vi "Navigation_Main_r2.2.vi"() -> ()   [LabVIEW 2015]
uses:
  <vilib>/myRIO/Instrument Drivers/Onboard IO/PWM/typedefs/PWM Reference.ctl
  <vilib>/myRIO/Common/Instrument Driver Framework/Utilities/typedefs/myRIO Generic Hardware Reference.ctl
  <vilib>/myRIO/Common/Instrument Driver Framework/Utilities/typedefs/Hardware Version Enum.ctl
  <vilib>/myRIO/Common/Instrument Driver Framework/Utilities/typedefs/myRIO v1.0 Reference.ctl
  <vilib>/myRIO/Common/Instrument Driver Framework/Utilities/typedefs/Generic FPGA Reference.ctl
  <vilib>/myRIO/Common/Instrument Driver Framework/myRIO v1.0/PWM/typedefs/PWM Channels Enum.ctl
  <vilib>/myRIO/Instrument Drivers/Onboard IO/PWM/typedefs/PWM Configuration.ctl
  <vilib>/userdefined/High Color/nirio_resource_hc.ctl
  <vilib>/myRIO/Common/Instrument Driver Framework/myRIO v1.0/PWM/vis/myRIO v1.1 Open PWM.vi
  <vilib>/myRIO/Common/Instrument Driver Framework/Utilities/vis/Validate Channels.vi
  <vilib>/myRIO/Common/Instrument Driver Framework/myRIO v1.0/PWM/vis/myRIO v1.0 Reserve PWM.vi
  <vilib>/myRIO/Common/Instrument Driver Framework/myRIO v1.0/PWM/vis/myRIO v1.0 Build MUX Configuration PWM.vi
  <vilib>/myRIO/Common/Instrument Driver Framework/myRIO v1.0/Resource Manager/vis/myRIO v1.0 Reserve Channel List.vi
  <vilib>/myRIO/Common/Instrument Driver Framework/myRIO v1.0/Resource Manager/vis/myRIO v1.0 Create Configuration List.vi
  <vilib>/myRIO/Common/Instrument Driver Framework/myRIO v1.0/Resource Manager/vis/myRIO v1.0 Reserve Channel.vi
  <vilib>/myRIO/Common/Instrument Driver Framework/myRIO v1.0/Resource Manager/vis/myRIO v1.0 Unreserve Channel.vi
  <vilib>/myRIO/Common/Instrument Driver Framework/myRIO v1.0/Resource Manager/vis/myRIO v1.0 Build Mutex Name.vi
  <vilib>/FPGAPlugInAG/myRIO-1900/niLvFpga_Open_myRIO-1900.vi
  <vilib>/rvi/interface/common/dynamic/niFpgaDynamicAddResources.vi
  <vilib>/myRIO/Common/Instrument Driver Framework/Utilities/vis/FPGA Ref Manager.vi
  <vilib>/Utility/error.llb/Error Cluster From Error Code.vi
  <vilib>/myRIO/Common/Instrument Driver Framework/Utilities/vis/Ref Counter.vi
  <vilib>/rvi/errors/niLvFpgaAdjustHostInterfaceError.vi
  <vilib>/Utility/VariantDataType/GetNumericInfo.vi
  <vilib>/myRIO/Common/Instrument Driver Framework/myRIO v1.0/myRIO v1.1 Open.vi
  <vilib>/myRIO/Common/Instrument Driver Framework/Utilities/vis/IO Manager.vi
  <vilib>/myRIO/Common/Instrument Driver Framework/Utilities/vis/Configuration Manager.vi
  <vilib>/myRIO/Common/Instrument Driver Framework/myRIO v1.0/Resource Manager/vis/myRIO v1.0 Configure IO.vi
  <vilib>/myRIO/Common/Instrument Driver Framework/myRIO v1.0/myRIO v1.0 Close.vi
  <vilib>/myRIO/Common/Instrument Driver Framework/myRIO v1.0/PWM/vis/myRIO v1.0 Write PWM.vi
  <vilib>/addons/control/pid/pid.llb/PID (DBL).vi
  <vilib>/rvi/interface/nirviOpenFPGA/nirviOpenFPGA.xnode
  Navi/E/FPGA Bitfiles/NavigationProjec_FPGATarget2_FPGAMainNavigati_PWPHW8gwDxI.lvbitx
  <vilib>/rvi/interface/nirviReadWriteControl/nirviReadWriteControl.xnode
  <vilib>/myRIO/Instrument Drivers/Onboard IO/PWM/vis/myRIO PWM Open.xnode
  <vilib>/myRIO/Instrument Drivers/Onboard IO/PWM/PWM.lvlib
  <vilib>/myRIO/Instrument Drivers/Utilities/Utilities.lvlib
  NiFpgaLv.dll
  <vilib>/rvi/interface/Simulation/niFpgaSimulationCallBeginRW.vi
  <vilib>/addons/control/pid/NI_PID_pid.lvlib
panel:
  out "Navigation\nCurrent \nAngle":dbl
  out "Navigation\nCurrent y\nPosition":dbl
  out "Navigation\nCurrent X\nPosition":dbl
  out "x+y":dbl
  out "angle command":dbl
  in  "y goal":dbl format="%#_13g"
  out "current angle":dbl
  in  "initial angle":dbl format="%#_13g"
  out "cout per foot":dbl
  out "x/y":dbl
  out "scale":dbl=1.0
  in  "x goal":dbl=10.0
  in  "L Desired Input Velocity (ft/s) 4":dbl(knob) scale=-4.0..4.0
  out "x position 5":dbl
  in  "R Desired Input Velocity (ft/s) 5":dbl(knob) scale=-4.0..4.0
  in  "R Desired Input Velocity (ft/s) 4":dbl(knob) scale=-4.0..4.0
  in  "L Desired Input Velocity (ft/s) 3":dbl(knob) scale=-4.0..4.0
  in  "R Desired Input Velocity (ft/s) 3":dbl(knob) scale=-4.0..4.0
  in  "L Desired Input Velocity (ft/s) 2":dbl(knob) scale=-4.0..4.0
  in  "R Desired Input Velocity (ft/s) 2":dbl(knob) scale=-4.0..4.0
  in  "L Desired Input Velocity (ft/s)":dbl(knob) scale=-4.0..4.0
  out "left":dbl
  out "right":dbl
  out "actual pwm 2":dbl
  in  "stop 3":bool
  out "left pwm":dbl(graph)
  out "dt out (s) 3":dbl format="%.3f"
  in  "output range 3":cluster{"output high":dbl, "output low":dbl}={"output high"=0.13333, "output low"=-0.13333} {"output low" format="%.6f"; "output high" format="%.5f"}
  in  "PID gains 3":T1={"proportional gain (Kc)"=0.002, "integral time (Ti, min)"=7e-07, "derivative time (Td, min)"=0.0} {"derivative time (Td, min)" format="%.8f"; "integral time (Ti, min)" format="%.8f"; "proportional gain (Kc)" format="%.8f"}
  out "desired pwm 2":dbl
  out "feedback 2":dbl
  out ".not. x? 3":bool
  out "Elapsed Time (s) 2":dbl caption="Elapsed Time (s)"
  out "x traveled 2":dbl
  out "y traveled 2":dbl
  out "avg right":dbl
  out "avg left":dbl
  out "psi dot":dbl
  out "distance traveled 2":dbl
  out "y dot 2":dbl
  out "x dot 2":dbl
  out "x position":dbl
  out "y position":dbl
  out "reset x y 2":dbl
  out "Tick Count(mSec) 2":u32 caption="Tick Count(mSec)"
  in  "start y 2":dbl=3.0
  in  "start x 2":dbl=1.0
  in  "start y":dbl=3.0
  in  "start x":dbl=1.0
  in  "Encoder Reset 2":bool
  out "actual pwm":dbl
  in  "stop 2":bool
  out "right pwm":dbl(graph)
  out "dt out (s) 2":dbl format="%.3f"
  in  "output range 2":cluster{"output high":dbl, "output low":dbl}={"output high"=0.13333, "output low"=-0.13333} {"output low" format="%.6f"; "output high" format="%.5f"}
  in  "PID gains 2":T1={"proportional gain (Kc)"=0.002, "integral time (Ti, min)"=7e-07, "derivative time (Td, min)"=0.0} {"derivative time (Td, min)" format="%.8f"; "integral time (Ti, min)" format="%.8f"; "proportional gain (Kc)" format="%.8f"}
  out "desired pwm":dbl
  out "feedback":dbl
  out ".not. x? 2":bool
  out "Elapsed Time (s)":dbl
  out "LF Rot Velocity (rot/s)":dbl
  out "LM Rot Velocity (rot/s)":dbl
  out "LR Rot Velocity (rot/s)":dbl
  out "RR Rot Velocity (rot/s)":dbl
  out "RM Linear Velocity (rot/s)":dbl
  out "RF Linear Velocity (rot/s)":dbl
  in  "Encoder Reset":bool
  out "SYS.SELECTA":u8 format="%08b"
  out "ENC.B_c.CNTR":i32
  out "ENC.B_b.CNTR":i32
  out "ENC.B_a.CNTR":i32
  out "ENC.A_c.CNTR":i32
  out "ENC.A_b.CNTR":i32
  out "ENC.A_a.CNTR":i32
  in  "R Min Linear Velocity (ft/s)":dbl=-2.0 format="%#_13g"
  in  "R Max Linear Velocity (ft/s)":dbl=2.0 format="%#_13g"
  in  "L Min Linear Velocity (ft/s)":dbl=-2.0 format="%#_13g"
  in  "L Max Linear Velocity (ft/s)":dbl=2.0 format="%#_13g"
  out "Current Rot Velocity (rot/s)":T2(graph)
  # "Motor Control Parameters"
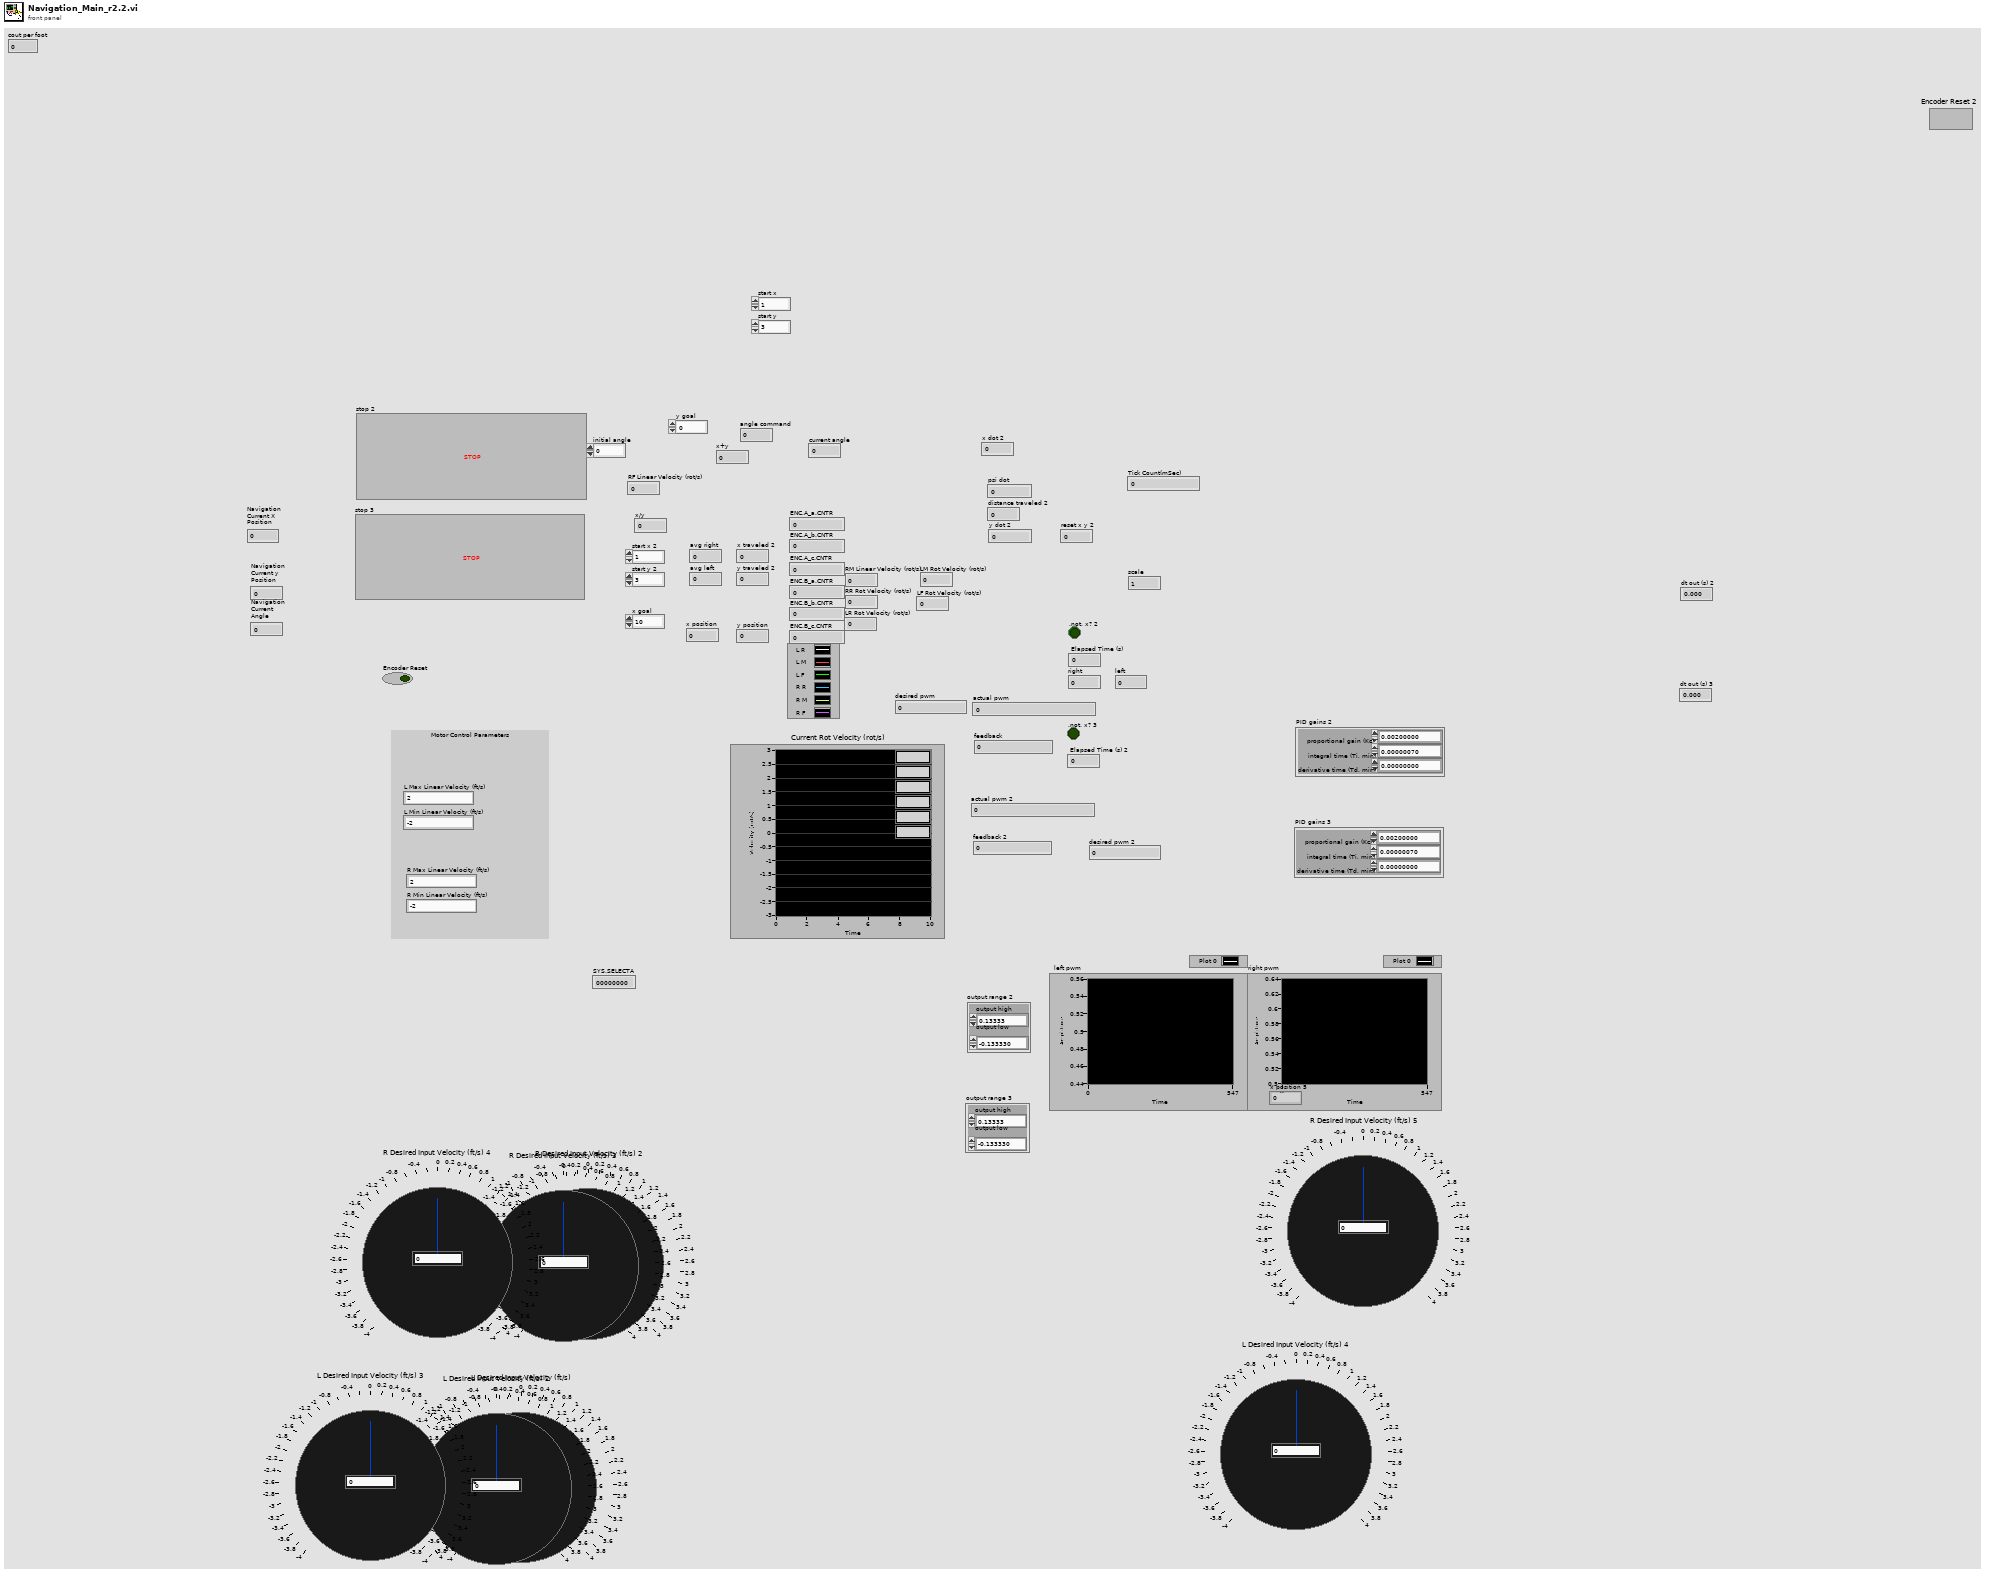
[diagram p1: front panel]
types:
  T1 = cluster{"proportional gain (Kc)":dbl, "integral time (Ti, min)":dbl, "derivative time (Td, min)":dbl}
  T2 = cluster{"Rotational Velocity (RPS)":dbl, "Rotational Velocity (RPS)":dbl, "Rotational Velocity (RPS)":dbl, "Rotational Velocity (RPS)":dbl, "Rotational Velocity (RPS)":dbl, "Rotational Velocity (RPS)":dbl}
  T3 = typedef "nirio_resource_hc.ctl" = tag
  T4 = typedef "Hardware Version Enum.ctl" = enum16{"Unknown", "myRIO-1900", "myRIO-1950", "roboRIO"}
  T5 = typedef "PWM.lvlib/PWM Reference.ctl" = cluster{"myRIO Reference":T6, "PWM Channels Enum":T9, "PWM Configuration":T10}
  T6 = typedef "myRIO Generic Hardware Reference.ctl" = cluster{"myRIO Model":T4, "myRIO Hardware Reference":T7}
  T7 = typedef "myRIO v1.0 Reference.ctl" = cluster{"Generic FPGA Reference":T8, "Allow multiple opens":bool}
  T8 = typedef "Generic FPGA Reference.ctl" = refnum<k20>
  T9 = typedef "PWM Channels Enum.ctl" = enum16{"Not Connected", "C/PWM0", "C/PWM1", "A/PWM0", "A/PWM1", "A/PWM2", "B/PWM0", "B/PWM1", "B/PWM2", "PWM/PWM0", "PWM/PWM1", "PWM/PWM2", "PWM/PWM3", "PWM/PWM4", "PWM/PWM5", "PWM/PWM6", "PWM/PWM7", "PWM/PWM8", "PWM/PWM9"}
  T10 = typedef "PWM.lvlib/PWM Configuration.ctl" = cluster{"Frequency":dbl, "Duty Cycle":dbl}
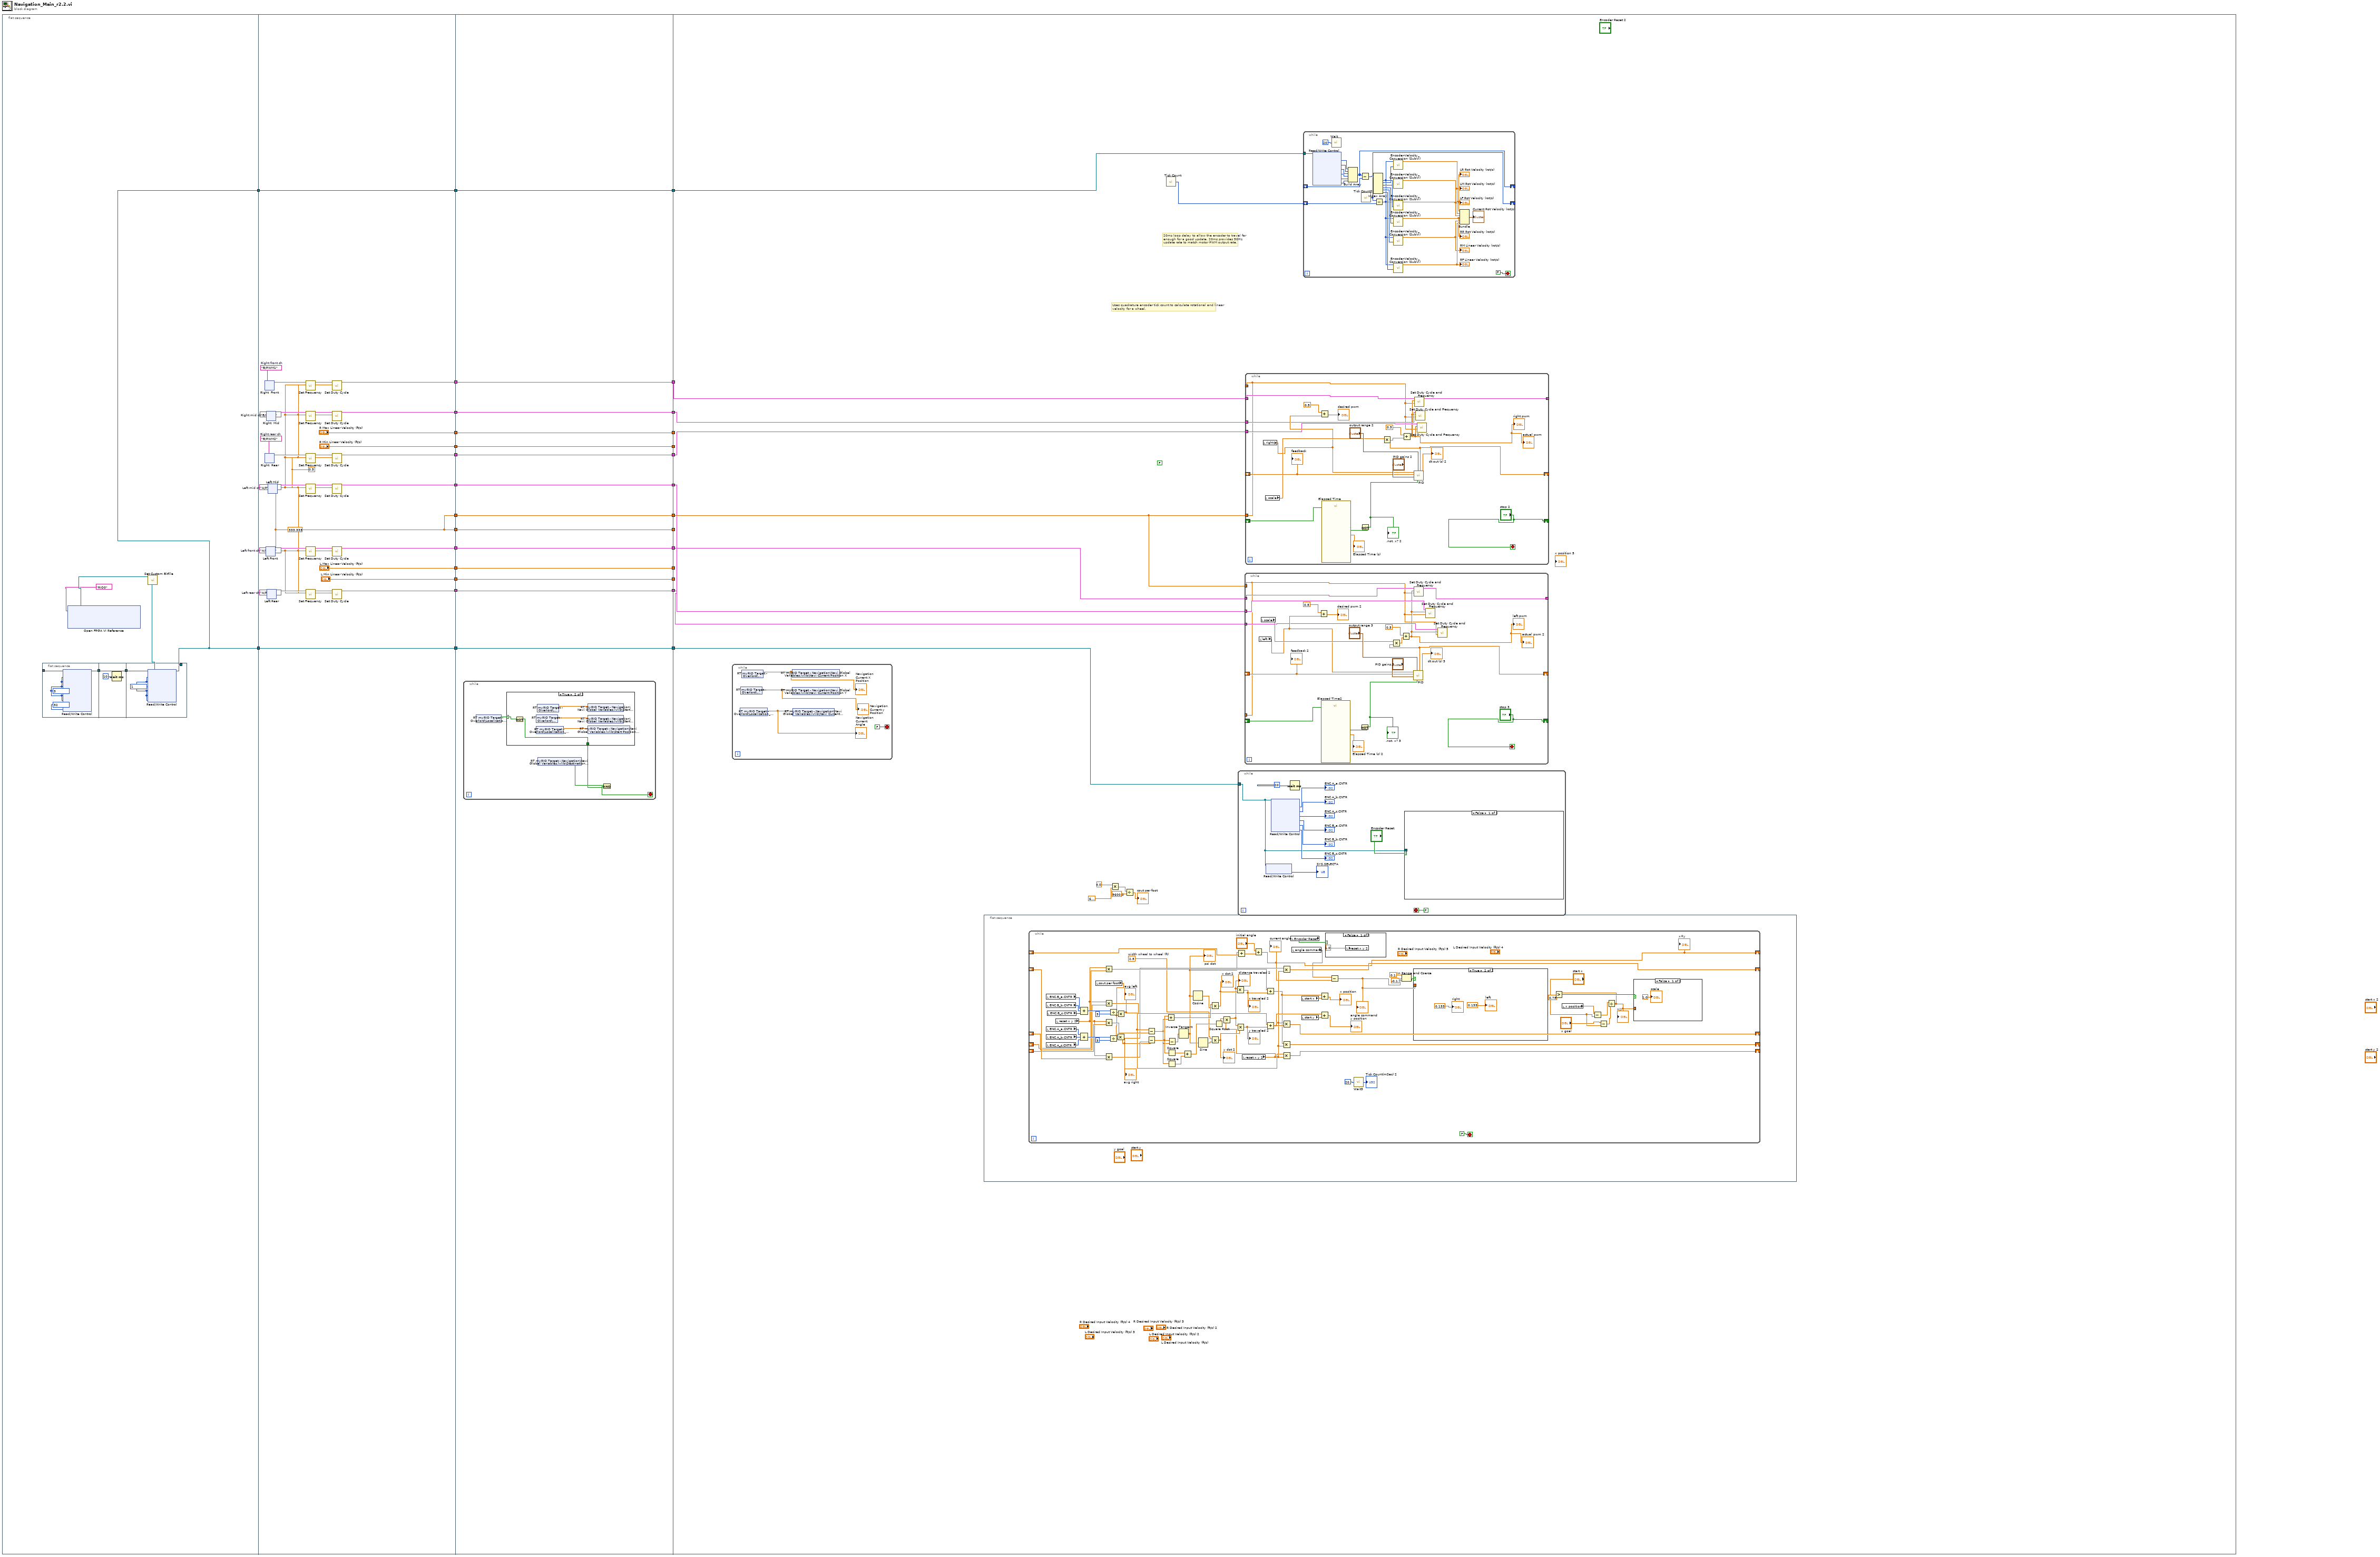
[diagram p0: block diagram]
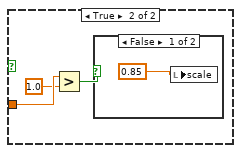
[diagram p3: hidden frame]
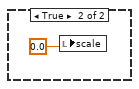
[diagram p4: hidden frame]
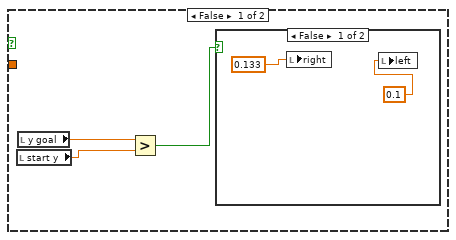
[diagram p5: hidden frame]
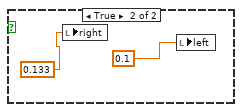
[diagram p6: hidden frame]
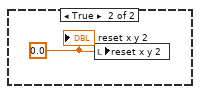
[diagram p7: hidden frame]
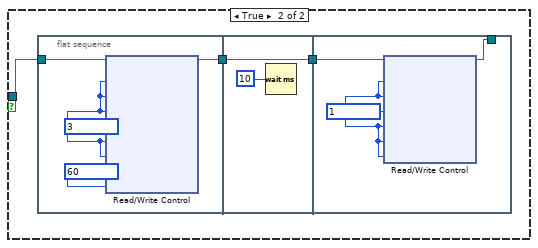
[diagram p8: hidden frame]
diagram:
  n1 = flat-sequence {
    tunnel: [w33] -> w30
    tunnel: [w33] -> w29
    tunnel: [w46] -> w28
    tunnel: [w61] -> w26
    tunnel: [w57] -> w24
    tunnel: [w56] -> w22
    tunnel: [w55] -> w20
    tunnel: [w54] -> w18
    tunnel: [w53] -> w16
    tunnel: ["L Max Linear Velocity (ft/s)"] -> w14
    tunnel: ["L Min Linear Velocity (ft/s)"] -> w12
    tunnel: ["R Max Linear Velocity (ft/s)"] -> w10
    tunnel: ["R Min Linear Velocity (ft/s)"] -> w8
    tunnel: [w48] -> w6
    tunnel: w30 -> [w47]
    tunnel: [w47] -> w4
    tunnel: w29 -> [w48]
    tunnel: [w46] -> w2
    tunnel: w28 -> [w187]
    tunnel: [w187] -> w27
    tunnel: w26 -> [w186]
    tunnel: [w186] -> w25
    tunnel: w24 -> [w185]
    tunnel: [w185] -> w23
    tunnel: w22 -> [w184]
    tunnel: [w184] -> w21
    tunnel: w20 -> [w183]
    tunnel: [w183] -> w19
    tunnel: w18 -> [w182]
    tunnel: [w182] -> w17
    tunnel: w16 -> [w181]
    tunnel: [w181] -> w15
    tunnel: w14 -> [w180]
    tunnel: [w180] -> w13
    tunnel: w12 -> [w179]
    tunnel: [w179] -> w11
    tunnel: w10 -> [w178]
    tunnel: [w178] -> w9
    tunnel: w8 -> [w177]
    tunnel: [w177] -> w7
    tunnel: w6 -> [w176]
    tunnel: [w176] -> w5
    tunnel: w4 -> [w175]
    tunnel: [w175] -> w3
    tunnel: w2 -> [w174]
    tunnel: [w174] -> w1
    tunnel: w27 -> [_]
    tunnel: w25 -> [w202]
    tunnel: w23 -> [w208]
    tunnel: w21 -> [w205]
    tunnel: w19 -> [w204]
    tunnel: w17 -> [w203]
    tunnel: w15 -> [w207]
    tunnel: w13 -> [_]
    tunnel: w11 -> [_]
    tunnel: w9 -> [_]
    tunnel: w7 -> [_]
    tunnel: w5 -> [w210]
    tunnel: w3 -> [w209]
    tunnel: w1 -> [w206]
    frame #0 {
      n2 = flat-sequence {
        tunnel: w34 -> [w39]
        tunnel: [w37] -> w36
        tunnel: w36 -> [w41]
        tunnel: [w41] -> w35
        tunnel: w35 -> [w44]
        tunnel: [w43] -> w33
        frame #0 {
          w38 = u8 32 ("SYS.SELECTA")
          w40 = u8 3 ("ENC.B_c.CNFG")
          n3 = xnode "Read/Write Control"("FPGA VI Reference In"=w39, "ENC.A_a.CNFG"=w40, "ENC.A_b.CNFG"=w40, "ENC.A_c.CNFG"=w40, "ENC.B_a.CNFG"=w40, "ENC.B_b.CNFG"=w40, "ENC.B_c.CNFG"=w40, "SYS.SELECTA"=w38, "SYS.SELECTB"=w38) -> ("FPGA VI Reference Out"=w37:refnum<k20>)  [unwired: 1 in, 1 out]
        }
        frame #1 {
          n4 = Wait (ms)(milliseconds to wait=u32 10) -> ()  [unwired: 1 out]
        }
        frame #2 {
          w45 = u8 1 ("ENC.B_c.CNFG")
          n5 = xnode "Read/Write Control"("FPGA VI Reference In"=w44, "ENC.A_a.CNFG"=w45, "ENC.A_b.CNFG"=w45, "ENC.A_c.CNFG"=w45, "ENC.B_a.CNFG"=w45, "ENC.B_b.CNFG"=w45, "ENC.B_c.CNFG"=w45) -> ("FPGA VI Reference Out"=w43:refnum<k20>)  [unwired: 1 in, 1 out]
        }
      }
      n6 = xnode "Open FPGA VI Reference"("resource name"=tag "RIO0") -> ("FPGA VI Reference Out"=w32:refnum<k20>)  [unwired: 1 in, 1 out]
      n7 = call <vilib>:"Set Custom Bitfile.vi"("Custom FPGA Reference In"=w32) -> ("Custom FPGA Reference Out"=w34:refnum<k20>)  [unwired: 9 in, 1 out]
    }
    frame #1 {
      w58 = 0.5 ("Duty Cycle")
      w46 = 333.333 ("Frequency [Hz]")
      w72 = tag "B/PWM2"  # Right rear ch
      w73 = tag "B/PWM0"  # Right mid ch
      w74 = tag "B/PWM1"  # Right front ch
      w75 = tag "A/PWM2"  # Left rear ch
      w76 = tag "A/PWM1"  # Left mid ch
      w77 = tag "A/PWM0"  # Left front ch
      n8 = xnode "Right  Front"("Channel Name"=w74) -> ("PWM Ref Out"=w68:T5)  [unwired: 2 in, 1 out]
      n9 = xnode "Right  Rear"("Channel Name"=w72) -> ("PWM Ref Out"=w66:T5)  [unwired: 2 in, 1 out]
      n10 = xnode "Left Front"("Channel Name"=w77) -> ("PWM Ref Out"=w71:T5)  [unwired: 2 in, 1 out]
      n11 = xnode "Right  Mid"("Channel Name"=w73) -> ("PWM Ref Out"=w67:T5)  [unwired: 2 in, 1 out]
      n12 = xnode "Left Rear"("Channel Name"=w75) -> ("PWM Ref Out"=w69:T5)  [unwired: 2 in, 1 out]
      n13 = xnode "Left Mid"("Channel Name"=w76) -> ("PWM Ref Out"=w70:T5)  [unwired: 2 in, 1 out]
      n14 = call <vilib>:"Set Frequency.vi"("Frequency [Hz]"=w46, "PWM Ref In"=w68) -> ("PWM Ref Out"=w62:T5)  [unwired: 7 in, 1 out]
      n15 = call <vilib>:"Set Frequency.vi"("Frequency [Hz]"=w46, "PWM Ref In"=w67) -> ("PWM Ref Out"=w63:T5)  [unwired: 7 in, 1 out]
      n16 = call <vilib>:"Set Frequency.vi"("Frequency [Hz]"=w46, "PWM Ref In"=w66) -> ("PWM Ref Out"=w64:T5)  [unwired: 7 in, 1 out]
      n17 = call <vilib>:"Set Frequency.vi"("Frequency [Hz]"=w46, "PWM Ref In"=w70) -> ("PWM Ref Out"=w59:T5)  [unwired: 7 in, 1 out]
      n18 = call <vilib>:"Set Frequency.vi"("Frequency [Hz]"=w46, "PWM Ref In"=w71) -> ("PWM Ref Out"=w65:T5)  [unwired: 7 in, 1 out]
      n19 = call <vilib>:"Set Frequency.vi"("Frequency [Hz]"=w46, "PWM Ref In"=w69) -> ("PWM Ref Out"=w60:T5)  [unwired: 7 in, 1 out]
      n20 = call <vilib>:"Set Duty Cycle.vi"("Duty Cycle"=w58, "PWM Ref In"=w62) -> ("PWM Ref Out"=w57:T5)  [unwired: 7 in, 1 out]
      n21 = call <vilib>:"Set Duty Cycle.vi"("Duty Cycle"=w58, "PWM Ref In"=w63) -> ("PWM Ref Out"=w56:T5)  [unwired: 7 in, 1 out]
      n22 = call <vilib>:"Set Duty Cycle.vi"("Duty Cycle"=w58, "PWM Ref In"=w64) -> ("PWM Ref Out"=w55:T5)  [unwired: 7 in, 1 out]
      n23 = call <vilib>:"Set Duty Cycle.vi"("Duty Cycle"=w58, "PWM Ref In"=w59) -> ("PWM Ref Out"=w54:T5)  [unwired: 7 in, 1 out]
      n24 = call <vilib>:"Set Duty Cycle.vi"("Duty Cycle"=w58, "PWM Ref In"=w65) -> ("PWM Ref Out"=w53:T5)  [unwired: 7 in, 1 out]
      n25 = call <vilib>:"Set Duty Cycle.vi"("Duty Cycle"=w58, "PWM Ref In"=w60) -> ("PWM Ref Out"=w61:T5)  [unwired: 7 in, 1 out]
    }
    frame #2 {
      n26 = while {
        stop <- w190 stop-if-true
        n27 = shared-variable "RT myRIO Target - Overlord\\Localization_Variables_r0.lvlib\\loc_flag"() -> (w189:bool)  [unwired: 1 in, 1 out]
        n28 = case shown="True" w189 {
          selector: w189 -> [_ w194]
          tunnel: [_ w193] -> w188
          frame False {
          }
          frame True {
            n29 = Not(x=w194) -> (.not. x?=w193:bool)
            n30 = shared-variable "RT myRIO Target - Overlord\\Localization_Variables_r0.lvlib\\loc_theta"() -> (w192:dbl)  [unwired: 1 in, 1 out]
            n31 = shared-variable "RT myRIO Target - Overlord\\Localization_Variables_r0.lvlib\\loc_y"() -> (w195:dbl)  [unwired: 1 in, 1 out]
            n32 = shared-variable "RT myRIO Target - Overlord\\Localization_Variables_r0.lvlib\\loc_x"() -> (w196:dbl)  [unwired: 1 in, 1 out]
            n33 = shared-variable "RT myRIO Target - Navigation\\Navi Global Variables.lvlib\\Start Position X"(w196) -> ()  [unwired: 1 in, 1 out]
            n34 = shared-variable "RT myRIO Target - Navigation\\Navi Global Variables.lvlib\\Start Position Y"(w195) -> ()  [unwired: 1 in, 1 out]
            n35 = shared-variable "RT myRIO Target - Navigation\\Navi Global Variables.lvlib\\Start Position Angle"(w192) -> ()  [unwired: 1 in, 1 out]
          }
        }
        n36 = shared-variable "RT myRIO Target - Navigation\\Navi Global Variables.lvlib\\Destination Reached"() -> (w191:bool)  [unwired: 1 in, 1 out]
        n37 = And(x=w191, y=w188) -> (x .and. y?=w190:bool)
      }
    }
    frame #3 {
      (unwired) FALSE
      # "Uses quadrature encoder tick count to calculate rotational and linear velocity for a wheel."
      # "20ms loop delay to allow the encoder to travel far enough for a good update. 20ms provides 50Hz update rate to match motor PWM output rate."
      n38 = while {
        stop <- FALSE stop-if-true
        n39 = shared-variable "RT myRIO Target - Overlord\\Localization_Variables_r0.lvlib\\loc_theta"() -> (w212:dbl)  [unwired: 1 in, 1 out]
        "Navigation\nCurrent \nAngle" <- w212
        n40 = shared-variable "RT myRIO Target - Overlord\\Localization_Variables_r0.lvlib\\loc_y"() -> (w213:dbl)  [unwired: 1 in, 1 out]
        "Navigation\nCurrent y\nPosition" <- w213
        n41 = shared-variable "RT myRIO Target - Overlord\\Localization_Variables_r0.lvlib\\loc_x"() -> (w214:dbl)  [unwired: 1 in, 1 out]
        "Navigation\nCurrent X\nPosition" <- w214
        n42 = shared-variable "RT myRIO Target - Navigation\\Navi Global Variables.lvlib\\Navi Current Position X"(w214) -> ()  [unwired: 1 in, 1 out]
        n43 = shared-variable "RT myRIO Target - Navigation\\Navi Global Variables.lvlib\\Navi Current Position Y"(w213) -> ()  [unwired: 1 in, 1 out]
        n44 = shared-variable "RT myRIO Target - Navigation\\Navi Global Variables.lvlib\\Navi Current Angle"(w212) -> ()  [unwired: 1 in, 1 out]
      }
      n45 = flat-sequence {
        frame #0 {
          n46 = while {
            shift-right: [w250] -> _
            shift-left: _ -> [w275]
            shift-right: [w247] -> _
            shift-left: _ -> [w274]
            shift-right: [w249] -> _
            shift-left: _ -> [w259]
            shift-right: [w248] -> _
            shift-left: _ -> [w258]
            shift-right: [w224] -> _
            shift-left: _ -> [w228]
            stop <- FALSE stop-if-true
            w221 = 2.5  # width wheel to wheel (ft)
            n47 = local read "ENC.B_a.CNTR"() -> (w280:i32)
            n48 = local read "ENC.B_b.CNTR"() -> (w279:i32)
            n49 = local read "ENC.A_a.CNTR"() -> (w283:i32)
            n50 = local read "ENC.A_b.CNTR"() -> (w282:i32)
            n51 = local read "ENC.A_c.CNTR"() -> (w281:i32)
            n52 = local read "ENC.B_c.CNTR"() -> (w278:i32)
            n53 = local read "reset x y 2"() -> (w246:dbl)
            n54 = Compound Arithmetic op=ADD(w280, w279, w278) -> (w286:i32)
            n55 = Compound Arithmetic op=ADD(w283, w282, w281) -> (w287:i32)
            n56 = local read "cout per foot"() -> (w229:dbl)
            n57 = Multiply(x=w246, y=w258) -> (x*y=w252:dbl)
            n58 = Multiply(x=w246, y=w259) -> (x*y=w253:dbl)
            n59 = Multiply(x=w246, y=w274) -> (x*y=w251:dbl)
            n60 = Multiply(x=w246, y=w275) -> (x*y=w254:dbl)
            n61 = Divide(x=w286, y=3) -> (x/y=w273:dbl)
            n62 = Divide(x=w287, y=3) -> (x/y=w276:dbl)
            n63 = Multiply(x=w229, y=w276) -> (x*y=w230:dbl)
            "avg right" <- w230
            n64 = Multiply(x=w273, y=w229) -> (x*y=w231:dbl)
            "avg left" <- w231
            n65 = Subtract(x=w231, y=w251) -> (x-y=w270:dbl)
            n66 = Subtract(x=w230, y=w254) -> (x-y=w271:dbl)
            n67 = Add(x=w271, y=w270) -> (x+y=w272:dbl)
            n68 = Square(x=w271) -> (x^2=w268:dbl)
            n69 = Square(x=w270) -> (x^2=w269:dbl)
            n70 = Subtract(x=w271, y=w270) -> (x-y=w220:dbl)
            n71 = Inverse Tangent(1:w220) -> (0:w225:dbl)
            "psi dot" <- w225
            n72 = Add(x=w268, y=w269) -> (x+y=w267:dbl)
            n73 = Cosine(x=w225) -> (cos(x)=w265:dbl)
            n74 = Sine(x=w225) -> (sin(x)=w266:dbl)
            n75 = Multiply(x=w272, y=w265) -> (x*y=w263:dbl)
            "x dot 2" <- w263
            n76 = Multiply(x=w221, y=w266) -> (x*y=w264:dbl)
            "y dot 2" <- w264
            n77 = Square Root(x=w267) -> (sqrt(x)=w262:dbl)
            n78 = Add(x=w225, y=w228) -> (x+y=w227:dbl)
            n79 = local read "reset x y 2"() -> (w244:dbl)
            n80 = Multiply(x=w262, y=w244) -> (x*y=w245:dbl)
            "distance traveled 2" <- w245
            n81 = Multiply(x=w245, y=w263) -> (x*y=w261:dbl)
            "x traveled 2" <- w261
            n82 = Multiply(x=w245, y=w264) -> (x*y=w260:dbl)
            "y traveled 2" <- w260
            n83 = Add(x="initial angle", y=w227) -> (x+y=w224:dbl)
            "current angle" <- w224
            "x+y" <- w224
            n84 = Add(x=w252, y=w261) -> (x+y=w223:dbl)
            n85 = Add(x=w253, y=w260) -> (x+y=w255:dbl)
            n86 = Multiply(x=w230, y=w244) -> (x*y=w250:dbl)
            n87 = Multiply(x=w244, y=w255) -> (x*y=w249:dbl)
            n88 = Multiply(x=w223, y=w244) -> (x*y=w248:dbl)
            n89 = Multiply(x=w231, y=w244) -> (x*y=w247:dbl)
            n90 = local read "Encoder Reset"() -> (w243:bool)
            n91 = local read "angle command"() -> (w222:dbl)
            n92 = local read "start x"() -> (w256:dbl)
            n93 = local read "start y"() -> (w257:dbl)
            n94 = Add(x=w223, y=w256) -> (x+y=→"x position":dbl)
            n95 = Add(x=w255, y=w257) -> (x+y=→"y position":dbl)
            n96 = case shown="False" w243 {
              frame False {
                n97 = local write "reset x y 2"(1.0) -> ()
              }
              frame True {
                w305 = 0.0
                n98 = local write "reset x y 2"(w305) -> ()
                "reset x y 2" <- w305
              }
            }
            n99 = Subtract(x=w222, y=w224) -> (x-y=w216:dbl)
            "angle command" <- w216
            n100 = call "Wait3"("Count(mSec)"=u32 20) -> ("Tick Count(mSec)"=→"Tick Count(mSec) 2":u32)
            n101 = In Range and Coerce(upper limit=0.1 ("y"), x=w216, lower limit=-0.1) -> (In Range?=w219:bool)  [unwired: 1 out]
            n102 = case shown="True" w219 {
              tunnel: w216 -> [_ _]
              frame False {
                n103 = local read "start y"() -> (w296:dbl)
                n104 = local read "y goal"() -> (w297:dbl)
                n105 = Greater?(x=w297, y=w296) -> (0:w295:bool)
                n106 = case shown="False" w295 {
                  frame False {
                    n107 = local write "right"(0.133) -> ()
                    n108 = local write "left"(0.1 ("left")) -> ()
                  }
                  frame True {
                    n109 = local write "right"(0.133) -> ()
                    n110 = local write "left"(0.1) -> ()
                  }
                }
              }
              frame True {
                "right" <- 0.133
                "left" <- 0.133
              }
            }
            n111 = local read "x position"() -> (w239:dbl)
            n112 = Subtract(x=w239, y="start x") -> (x-y=w233:dbl)
            n113 = Subtract(x="x goal", y="start x") -> (x-y=w232:dbl)
            n114 = Divide(x=w233, y=w232) -> (x/y=w236:dbl)
            "x/y" <- w236
            n115 = Greater?(x=w236, y=0.75) -> (0:w237:bool)
            n116 = case shown="False" w237 {
              tunnel: w236 -> [_ w292]
              frame False {
                "scale" <- 1.0
              }
              frame True {
                n117 = Greater?(x=w292, y=1.0) -> (0:w290:bool)
                n118 = case shown="False" w290 {
                  frame False {
                    n119 = local write "scale"(0.85) -> ()
                  }
                  frame True {
                    n120 = local write "scale"(0.0) -> ()
                  }
                }
              }
            }
          }
        }
      }
      n121 = Multiply(x=4.0, y=6.283185307179586) -> (x*y=w197:dbl)
      n122 = Divide(x=w197, y=9600.0) -> (x/y=→"cout per foot":dbl)
      n123 = call "Tick Count"() -> ("Tick Count(uSec)"=w211:u32)
      n124 = while {
        tunnel: w210 -> [w350]
        stop <- FALSE stop-if-true
        n125 = xnode "Read/Write Control"("FPGA VI Reference In"=w350) -> ("SYS.SELECTA"=→"SYS.SELECTA":u8)  [unwired: 1 in, 2 out]
        n126 = xnode "Read/Write Control"("FPGA VI Reference In"=w350) -> ("ENC.A_a.CNTR"=→"ENC.A_a.CNTR":u32, "ENC.A_b.CNTR"=→"ENC.A_b.CNTR":u32, "ENC.A_c.CNTR"=→"ENC.A_c.CNTR":u32, "ENC.B_a.CNTR"=→"ENC.B_a.CNTR":u32, "ENC.B_b.CNTR"=→"ENC.B_b.CNTR":u32, "ENC.B_c.CNTR"=→"ENC.B_c.CNTR":u32)  [unwired: 1 in, 2 out]
        n127 = Wait (ms)(milliseconds to wait=u32 20) -> ()  [unwired: 1 out]
        n128 = case shown="False" "Encoder Reset" {
          tunnel: w350 -> [_ w361]
          frame False {
          }
          frame True {
            n129 = flat-sequence {
              tunnel: w361 -> [w366]
              tunnel: [w364] -> w363
              tunnel: w363 -> [w368]
              tunnel: [w368] -> w362
              tunnel: w362 -> [w371]
              tunnel: [w370] -> _
              frame #0 {
                w365 = u8 60 ("SYS.SELECTA")
                w367 = u8 3 ("ENC.B_c.CNFG")
                n130 = xnode "Read/Write Control"("FPGA VI Reference In"=w366, "ENC.A_a.CNFG"=w367, "ENC.A_b.CNFG"=w367, "ENC.A_c.CNFG"=w367, "ENC.B_a.CNFG"=w367, "ENC.B_b.CNFG"=w367, "ENC.B_c.CNFG"=w367, "SYS.SELECTA"=w365, "SYS.SELECTB"=w365) -> ("FPGA VI Reference Out"=w364:refnum<k20>)  [unwired: 1 in, 1 out]
              }
              frame #1 {
                n131 = Wait (ms)(milliseconds to wait=u32 10) -> ()  [unwired: 1 out]
              }
              frame #2 {
                w372 = u8 1 ("ENC.B_c.CNFG")
                n132 = xnode "Read/Write Control"("FPGA VI Reference In"=w371, "ENC.A_a.CNFG"=w372, "ENC.A_b.CNFG"=w372, "ENC.A_c.CNFG"=w372, "ENC.B_a.CNFG"=w372, "ENC.B_b.CNFG"=w372, "ENC.B_c.CNFG"=w372) -> ("FPGA VI Reference Out"=w370:refnum<k20>)  [unwired: 1 in, 1 out]
              }
            }
          }
        }
      }
      n133 = while {
        tunnel: w207 -> [w326]
        tunnel: [w327] -> _
        tunnel: w206 -> [w306]
        shift-right: [w312] -> _
        shift-left: _ -> [w322]
        shift-right: ["stop 3"] -> _
        shift-left: _ -> [w317]
        tunnel: [w306] -> _
        tunnel: w203 -> [w309]
        tunnel: w202 -> [w308]
        stop <- "stop 3" stop-if-true
        n134 = local read "left"() -> (w310:dbl)
        n135 = local read "scale"() -> (w313:dbl)
        n136 = Add(x=0.5, y=w310) -> (x+y=→"desired pwm 2":dbl)
        n137 = call "Elapsed Time2"("Reset"=w317) -> ("Elapsed Time (s)"=→"Elapsed Time (s) 2":dbl, "Time has Elapsed"=w320:bool)  [unwired: 11 in, 6 out]
        n138 = Not(x=w320) -> (.not. x?=w319:bool)
        ".not. x? 3" <- w319
        n139 = call-poly <vilib>:"PID.vi"("reinitialize? (F)"=w319, "output range"="output range 3", "PID gains"="PID gains 3", "process variable"=w322, "setpoint"=w310) -> ("dt out (s)"=→"dt out (s) 3":dbl, "output"=w312:dbl)  [unwired: 5 in]
        n140 = Multiply(x=w313, y=w312) -> (x*y=w311:dbl)
        n141 = Add(x=0.5, y=w311) -> (x+y=w307:dbl)
        "actual pwm 2" <- w307
        "left pwm" <- w307
        n142 = call <vilib>:"Set Duty Cycle and Frequency.vi"("Frequency [Hz]"=w306, "Duty Cycle"=w307, "PWM Ref In"=w326) -> ("PWM Ref Out"=w327:T5)  [unwired: 6 in, 1 out]
        n143 = call <vilib>:"Set Duty Cycle and Frequency.vi"("Frequency [Hz]"=w306, "Duty Cycle"=w307, "PWM Ref In"=w309) -> ()  [unwired: 6 in, 2 out]
        n144 = call <vilib>:"Set Duty Cycle and Frequency.vi"("Frequency [Hz]"=w306, "Duty Cycle"=w307, "PWM Ref In"=w308) -> ()  [unwired: 6 in, 2 out]
        "feedback 2" <- w322
      }
      n145 = while {
        tunnel: w208 -> [w348]
        tunnel: [w349] -> _
        tunnel: [w328] -> _
        shift-right: [w334] -> _
        shift-left: _ -> [w344]
        shift-right: ["stop 2"] -> _
        shift-left: _ -> [w339]
        tunnel: w206 -> [w328]
        tunnel: w205 -> [w331]
        tunnel: w204 -> [w330]
        stop <- "stop 2" stop-if-true
        n146 = local read "right"() -> (w332:dbl)
        n147 = local read "scale"() -> (w335:dbl)
        n148 = Add(x=0.5, y=w332) -> (x+y=→"desired pwm":dbl)
        n149 = call "Elapsed Time"("Reset"=w339) -> ("Elapsed Time (s)"=→"Elapsed Time (s)":dbl, "Time has Elapsed"=w342:bool)  [unwired: 11 in, 6 out]
        n150 = Not(x=w342) -> (.not. x?=w341:bool)
        ".not. x? 2" <- w341
        n151 = call-poly <vilib>:"PID.vi"("reinitialize? (F)"=w341, "output range"="output range 2", "PID gains"="PID gains 2", "process variable"=w344, "setpoint"=w332) -> ("dt out (s)"=→"dt out (s) 2":dbl, "output"=w334:dbl)  [unwired: 5 in]
        n152 = Multiply(x=w335, y=w334) -> (x*y=w333:dbl)
        n153 = Add(x=0.5, y=w333) -> (x+y=w329:dbl)
        "actual pwm" <- w329
        "right pwm" <- w329
        n154 = call <vilib>:"Set Duty Cycle and Frequency.vi"("Frequency [Hz]"=w328, "Duty Cycle"=w329, "PWM Ref In"=w348) -> ("PWM Ref Out"=w349:T5)  [unwired: 6 in, 1 out]
        n155 = call <vilib>:"Set Duty Cycle and Frequency.vi"("Frequency [Hz]"=w328, "Duty Cycle"=w329, "PWM Ref In"=w331) -> ()  [unwired: 6 in, 2 out]
        n156 = call <vilib>:"Set Duty Cycle and Frequency.vi"("Frequency [Hz]"=w328, "Duty Cycle"=w329, "PWM Ref In"=w330) -> ()  [unwired: 6 in, 2 out]
        "feedback" <- w344
      }
      n157 = while {
        shift-right: [w391] -> _
        shift-left: _ -> [w390]
        shift-right: [w388] -> _
        shift-left: w211 -> [w387]
        tunnel: w209 -> [w398]
        stop <- FALSE stop-if-true
        n158 = xnode "Read/Write Control"("FPGA VI Reference In"=w398) -> ("ENC.A_a.CNTR"=w397:u32, "ENC.A_b.CNTR"=w396:u32, "ENC.A_c.CNTR"=w395:u32, "ENC.B_a.CNTR"=w394:u32, "ENC.B_b.CNTR"=w393:u32, "ENC.B_c.CNTR"=w392:u32)  [unwired: 1 in, 2 out]
        n159 = call "Wait"("Count(mSec)"=u32 20) -> ()  [unwired: 1 out]
        n160 = Build Array(w397, w396, w395, w394, w393, w392) -> (w391:u32[])
        n161 = Subtract(x=w391, y=w390) -> (x-y=w389:u32[])
        n162 = call "Tick Count2"() -> ("Tick Count(uSec)"=w388:u32)
        n163 = Index Array(array=w389) -> (element #1=w386:u32, element #2=w385:u32, element #3=w384:u32, element #4=w383:u32, element #5=w382:u32, element #6=w381:u32)  [unwired: 6 in]
        n164 = Subtract(x=w388, y=w387) -> (x-y=w380:u32)
        n165 = call "Encoder-Velocity_Conversion (SubVI).vi"("delta  Encoder Count"=w385, "dt (uSec)"=w380) -> ("Rotational Velocity (RPS)"=w375:dbl)  [unwired: 7 in, 2 out]
        "LM Rot Velocity (rot/s)" <- w375
        n166 = call "Encoder-Velocity_Conversion (SubVI).vi"("delta  Encoder Count"=w384, "dt (uSec)"=w380) -> ("Rotational Velocity (RPS)"=w374:dbl)  [unwired: 7 in, 2 out]
        "LF Rot Velocity (rot/s)" <- w374
        n167 = call "Encoder-Velocity_Conversion (SubVI).vi"("delta  Encoder Count"=w386, "dt (uSec)"=w380) -> ("Rotational Velocity (RPS)"=w376:dbl)  [unwired: 7 in, 2 out]
        "LR Rot Velocity (rot/s)" <- w376
        n168 = call "Encoder-Velocity_Conversion (SubVI).vi"("delta  Encoder Count"=w383, "dt (uSec)"=w380) -> ("Rotational Velocity (RPS)"=w373:dbl)  [unwired: 7 in, 2 out]
        "RR Rot Velocity (rot/s)" <- w373
        n169 = call "Encoder-Velocity_Conversion (SubVI).vi"("delta  Encoder Count"=w382, "dt (uSec)"=w380) -> ("Rotational Velocity (RPS)"=w377:dbl)  [unwired: 7 in, 2 out]
        "RM Linear Velocity (rot/s)" <- w377
        n170 = call "Encoder-Velocity_Conversion (SubVI).vi"("delta  Encoder Count"=w381, "dt (uSec)"=w380) -> ("Rotational Velocity (RPS)"=w378:dbl)  [unwired: 7 in, 2 out]
        "RF Linear Velocity (rot/s)" <- w378
        n171 = Bundle("Rotational Velocity (RPS)"=w376, "Rotational Velocity (RPS)"=w375, "Rotational Velocity (RPS)"=w374, "Rotational Velocity (RPS)"=w373, "Rotational Velocity (RPS)"=w377, "Rotational Velocity (RPS)"=w378) -> (→"Current Rot Velocity (rot/s)":T2)  [unwired: 1 in]
      }
    }
  }
